vi "MakeTableItem_Init.vi"(8 "error in (no error)":errorcluster, 10 "Item":T1, 11 "object in":refnum<class "ConcreteTableItem.lvclass">) -> (0 "error out":errorcluster, 3 "object out":refnum<class "ConcreteTableItem.lvclass">)   [LabVIEW 2015, in "ActorManagement.lvlib" / "ConcreteTableItem.lvclass"]
uses:
  ConcreteTableItem.lvclass
  ConcreteTableItem.lvclass/ConcreteTableItem.ctl
  Config/g_tabSetting.vi
  TableItem/TableItem.lvclass
  ActorManagement.lvlib
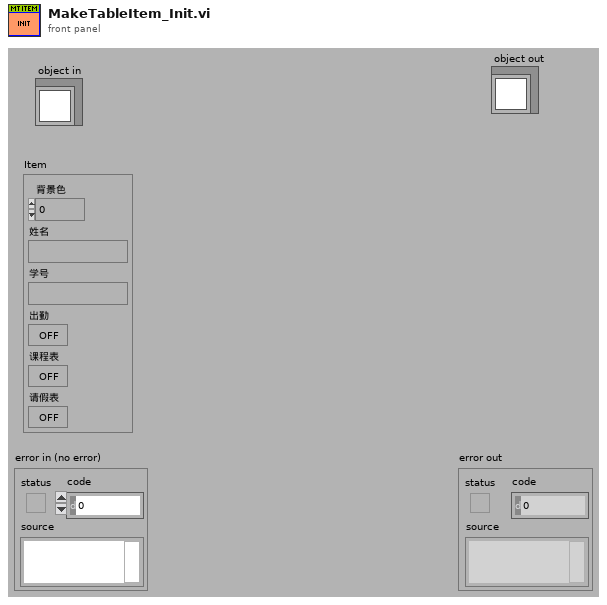
[diagram p1: front panel]
types:
  T1 = cluster{"背景色":u32, "姓名":string, "学号":string, "出勤":bool, "课程表":bool, "请假表":bool}
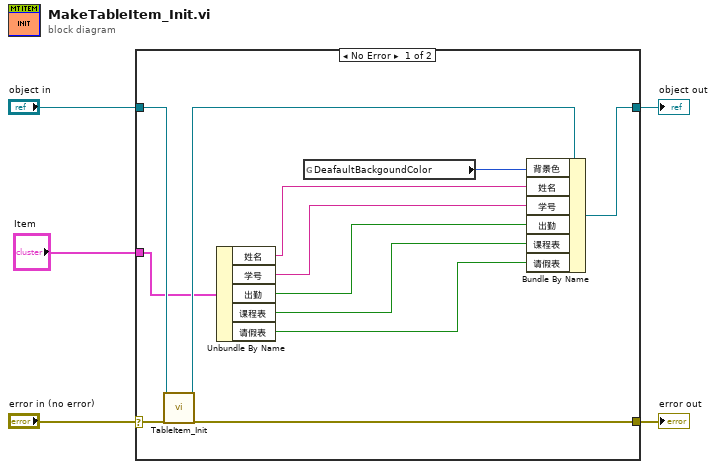
[diagram p0: block diagram]
diagram:
  n1 = case shown="No Error" "error in (no error)" {
    selector: "error in (no error)" -> [w16 w18]
    tunnel: [w17 w19] -> w5
    tunnel: "object in" -> [w14 w19]
    tunnel: [w15 w18] -> w2
    tunnel: "Item" -> [w11 _]
    frame No Error {
      n2 = call "TableItem_Init.vi"("object in"=w14, "error in (no error)"=w16) -> ("object out"=w13:refnum<class "ConcreteTableItem.lvclass">, "error out"=w15:errorcluster)  [unwired: 16 in]
      n3 = Unbundle By Name(w11) -> ("姓名"=w10:string, "学号"=w9:string, "出勤"=w8:bool, "课程表"=w7:bool, "请假表"=w6:bool)
      n4 = global read "g_tabSetting.vi" "DeafaultBackgoundColor"() -> (w12:u32)
      n5 = Bundle By Name(cluster=w13, "背景色"=w12, "姓名"=w10, "学号"=w9, "出勤"=w8, "课程表"=w7, "请假表"=w6) -> (w17:refnum<class "ConcreteTableItem.lvclass">)
    }
    frame Error {
    }
  }
  "object out" <- w5
  "error out" <- w2
